vi "propatinodo.vi"() -> ()   [LabVIEW 2018]
panel:
  out "数値 3":dbl
  in  "数値 2":dbl
  in  "数値":dbl
  in  "クラスタ":cluster{"ブール":bool, "ブール 2":bool}
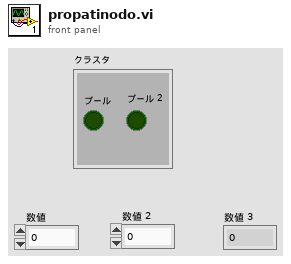
[diagram p1: front panel]
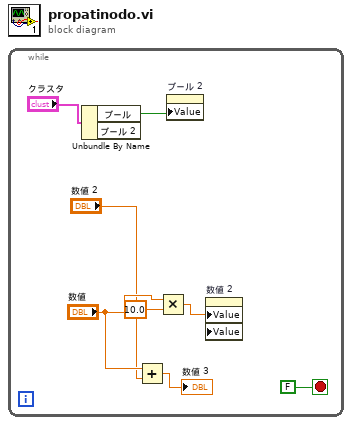
[diagram p0: block diagram]
diagram:
  n1 = while {
    stop <- FALSE stop-if-true
    n2 = Unbundle By Name("クラスタ") -> ("ブール"=w7:bool)  [unwired: 1 out]
    n3 = Add(x="数値", y="数値 2") -> (x+y=→"数値 3":dbl)
    n4 = Multiply(x="数値", y=10.0) -> (x*y=w4:dbl)
    n5 = property on="ブール 2" class="Bool (指定)"("Value"=w7) -> ()  [unwired: 2 in, 2 out]
    n6 = property on="数値 2" class="DigNum (指定)" props=["Value", "Value"]("Value"=w4) -> ()  [unwired: 3 in, 2 out]
  }
